vi "Untitled 12 (SubVI).vi"(0 "Subscriber list 2":string, 1 "Device Name (h)":refnum<vi>, 2 "shotnumber":refnum<vi>) -> ()   [LabVIEW 2009]
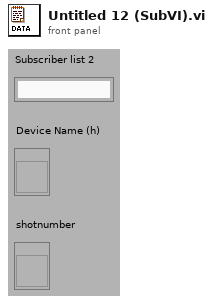
[diagram p1: front panel]
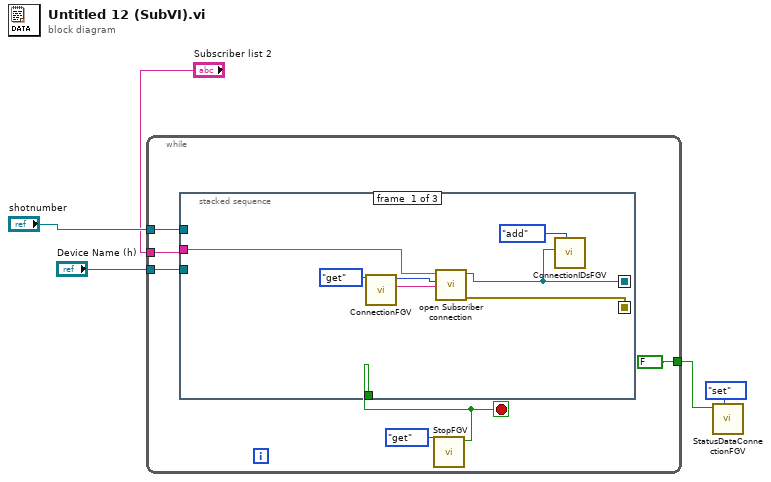
[diagram p0: block diagram]
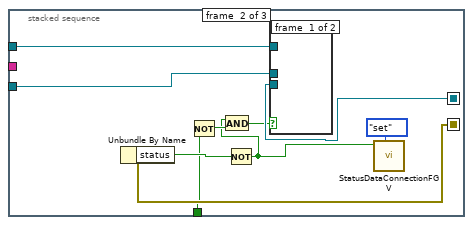
[diagram p2: hidden frame]
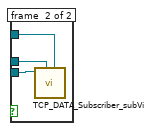
[diagram p3: hidden frame]
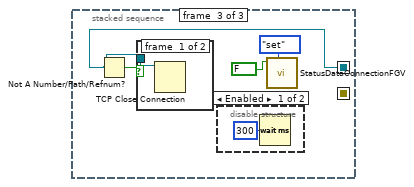
[diagram p4: hidden frame]
diagram:
  n1 = while {
    tunnel: [FALSE] -> w3
    tunnel: "Subscriber list 2" -> [w10]
    tunnel: "shotnumber" -> [w7]
    tunnel: "Device Name (h)" -> [w6]
    stop <- w8 stop-if-true
    n2 = call "StopFGV.vi"("Command"=enum16{"set", "get", "init"}."get") -> ("Stop out"=w8:bool)  [unwired: 10 in]
    n3 = stacked-sequence {
      seq-local: [w12 _ _] -> [_ w28 w34]
      seq-local: [w18 _ _] -> [_ w27 _]
      tunnel: w8 -> [_ w24 _]
      tunnel: w10 -> [w14 _ _]
      tunnel: w7 -> [_ w20 _]
      tunnel: w6 -> [_ w19 _]
      frame #0 {
        n4 = call "ConnectionFGV.vi"("command"=enum16{"get", "set", "init"}."get") -> ("Remote Host out"=w15:string, "port or service name out"=w16:u16)  [unwired: 9 in]
        n5 = call "open Subscriber connection.vi"("Machine"=w15, "Port"=w16, "Subscriber list"=w14) -> ("error out"=w18:errorcluster, "connection ID"=w12:refnum<k5>)  [unwired: 3 in]
        n6 = call "ConnectionIDsFGV.vi"("Command"=enum16{"add", "get", "init"}."add", "connection ID"=w12) -> ()  [unwired: 9 in, 1 out]
      }
      frame #1 {
        n7 = Unbundle By Name(w27) -> ("status"=w26:bool)
        n8 = Not(x=w24) -> (.not. x?=w25:bool)
        n9 = Not(x=w26) -> (.not. x?=w22:bool)
        n10 = And(x=w22, y=w25) -> (x .and. y?=w23:bool)
        n11 = case shown="True" w23 {
          tunnel: w28 -> [_ w31]
          tunnel: w20 -> [_ w30]
          tunnel: w19 -> [_ w29]
          frame #0 {
          }
          frame #1 {
            n12 = call "TCP_DATA_Subscriber_subVi.vi"("shot number"=w30, "whatamI"=w29, "connection ID"=w31) -> ()  [unwired: 8 in, 1 out]
          }
        }
        n13 = call "StatusDataConnectionFGV.vi"("Command"=enum16{"get", "set", "init"}."set", "Data Connection"=w22) -> ()  [unwired: 9 in, 1 out]
      }
      frame #2 {
        n14 = Not A Number/Path/Refnum?(number/path/refnum=w34) -> (NaN/Path/Refnum?=w35:bool)
        n15 = case shown="False" w35 {
          tunnel: w34 -> [w37 _]
          frame #0 {
            n16 = TCP Close Connection(connection ID=w37) -> ()  [unwired: 2 in, 2 out]
          }
          frame #1 {
          }
        }
        n17 = disable-structure shown="Enabled" {
          frame #0 {
            n18 = Wait (ms)(milliseconds to wait=u32 300 ("millisecond multiple")) -> ()  [unwired: 1 out]
          }
          frame #1 {
          }
        }
        n19 = call "StatusDataConnectionFGV.vi"("Command"=enum16{"get", "set", "init"}."set", "Data Connection"=FALSE ("status 2")) -> ()  [unwired: 9 in, 1 out]
      }
    }
  }
  n20 = call "StatusDataConnectionFGV.vi"("Command"=enum16{"get", "set", "init"}."set", "Data Connection"=w3) -> ()  [unwired: 9 in, 1 out]
